vi "PC vectornav input.vi"(10 "VISA resource name":refnum<visa-resource-name>="COM4") -> ()   [LabVIEW 2010]
uses:
  <vilib>/Instr/_visa.llb/VISA Configure Serial Port (Instr).vi
  UDP3-GPS, INS/UDP3GLOB.vi
  vectornav data.vi
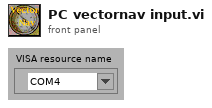
[diagram p1: front panel]
types:
  T1 = typedef "UDP 3.ctl" = cluster{"GPS":cluster{"Lat":dbl, "Longe":dbl}, "INS":cluster{"Heading":dbl, "x-magnetic":dbl, "y-magnetic":dbl, "z-magnetic":dbl, "x-acceleration":dbl, "y-acceleration":dbl, "z-acceleration":dbl}}
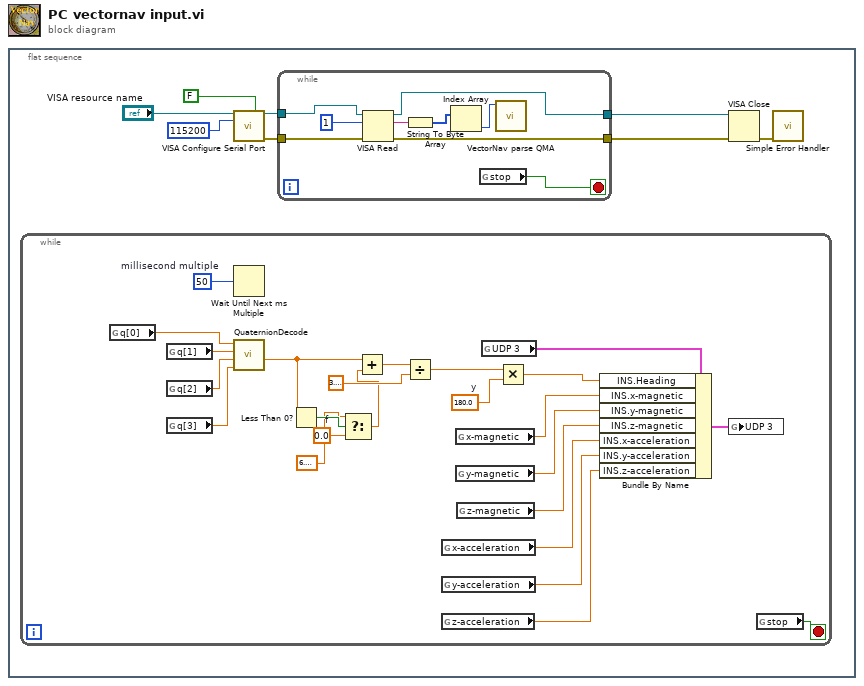
[diagram p0: block diagram]
diagram:
  n1 = flat-sequence {
    frame #0 {
      n2 = while {
        stop <- w15 stop-if-true
        w10 = 0.0  # f
        w17 = 180.0  # y
        w26 = u32 50  # millisecond multiple
        n3 = global read "vectornav data.vi" "q[0]"() -> (w25:dbl)
        n4 = global read "vectornav data.vi" "q[1]"() -> (w24:dbl)
        n5 = global read "vectornav data.vi" "q[2]"() -> (w23:dbl)
        n6 = global read "vectornav data.vi" "q[3]"() -> (w22:dbl)
        n7 = Wait Until Next ms Multiple(millisecond multiple=w26) -> ()  [unwired: 1 out]
        n8 = call "QuaternionDecode.vi"("qw"=w22, "qz"=w23, "qy"=w24, "qx"=w25) -> ("heading"=w13:dbl)  [unwired: 7 in]
        n9 = Less Than 0?(x=w13) -> (x < 0?=w12:bool)
        n10 = Select(t=6.283185307179586, s=w12, f=w10) -> (s? t:f=w9:dbl)
        n11 = Add(x=w13, y=w9) -> (x+y=w19:dbl)
        n12 = Divide(x=w19, y=3.141592653589793) -> (x/y=w18:dbl)
        n13 = global read "vectornav data.vi" "x-acceleration"() -> (w29:dbl)
        n14 = global read "vectornav data.vi" "y-acceleration"() -> (w28:dbl)
        n15 = global read "vectornav data.vi" "z-acceleration"() -> (w27:dbl)
        n16 = global read "vectornav data.vi" "x-magnetic"() -> (w32:dbl)
        n17 = global read "vectornav data.vi" "y-magnetic"() -> (w31:dbl)
        n18 = global read "vectornav data.vi" "z-magnetic"() -> (w30:dbl)
        n19 = global read "UDP3GLOB.vi" "UDP 3"() -> (w14:T1)
        n20 = Multiply(x=w18, y=w17) -> (x*y=w16:dbl)
        n21 = Bundle By Name(cluster=w14, "INS.Heading"=w16, "INS.x-magnetic"=w32, "INS.y-magnetic"=w31, "INS.z-magnetic"=w30, "INS.x-acceleration"=w29, "INS.y-acceleration"=w28, "INS.z-acceleration"=w27) -> (w21:T1)
        n22 = global write "UDP3GLOB.vi" "UDP 3"(w21) -> ()
        n23 = global read "UDP3GLOB.vi" "stop"() -> (w15:bool)
      }
      n24 = call-poly "VISA Configure Serial Port"("VISA resource name"="VISA resource name", "Enable Termination\nChar (T)"=FALSE ("Enable Termination\nChar (T)"), "baud rate (9600)"=u32 115200) -> ("VISA resource name out"=w5:refnum<visa-resource-name>, "error out"=w4:errorcluster)  [unwired: 6 in, 5 out]
      n25 = while {
        tunnel: w5 -> [w41]
        tunnel: w4 -> [w39]
        tunnel: [w38] -> w1
        tunnel: [w37] -> w2
        stop <- w34 stop-if-true
        n26 = VISA Read(VISA resource name=w41, byte count=u32 1, error in (no error)=w39) -> (VISA resource name out=w38:refnum<visa-resource-name>, read buffer=w36:string, error out=w37:errorcluster)  [unwired: 1 out]
        n27 = String To Byte Array(string=w36) -> (unsigned byte array=w35:u8[])
        n28 = Index Array(array=w35) -> (element=w33:u8)  [unwired: 1 in]
        n29 = global read "UDP3GLOB.vi" "stop"() -> (w34:bool)
        n30 = call "VectorNav parse QMA.vi"("input data"=w33) -> ()  [unwired: 11 in]
      }
      n31 = VISA Close(VISA resource name=w1, error in (no error)=w2) -> (error out=w3:errorcluster)
      n32 = call <vilib>:"Simple Error Handler.vi"("error in (no error)"=w3) -> ()  [unwired: 1 in, 8 out]
    }
  }
